vi "UHR-Fleezers Control (host) -Leonardo 04-2018 V4_fish.vi"(0 "Tab Green FB":T5(tab)=enum."Trap Control (RF)") -> ()   [LabVIEW 2014] (continued)
  n85 = xnode "Read/Write Control"("FPGA VI Reference In"=w153, "error in"=w173, "ai count"="AI Count (ticks)", "Interlace ON/OFF"=w139, "Number Interlace Cycles"=w138, "Set 1"=w19, "Set 2"=w18, "Set 3"=w17, "FB On/Off Set 1"=w260, "FB On/Off Set 2"=w259, "Interlace Off Parameters"=w137, "FB Setpoint Set 1"=w251, "FB Setpoint Set 2"=w250, "FB Gains"="PID gains", "FB output range"=cluster{"output high":i16, "output low":i16} {"output high"=3000, "output low"=0} ("FB output range 1"), "Cycles per step"=w236, "Scan BD"=w248, "Number of scans"=w232, "Scan steps"=w237, "Scan freq.  increment"=w238, "AO1 (Y)"=w220, "AO2 (X)"=w219, "Scan freq.  increment (MCL)"=w213, "Scan steps (MCL)"=w212, "Cycles per step (MCL)"=w211, "Number of scans (MCL)"=w210, "MCL count"=w136, "Cont. Scan (MCL)"=w209, "MCL Scan Axis"=w203, "1D or 2D Scan?"=w156, "N of AI1 Int Acq Sets"=w193, "BD 1 Delay (ticks)"="Freq switch delay", "Amp switch delay"="Amp switch delay", "Swap F1 and F2"="Swap F1 and F2", "APD Acq Rate Count"=w161, "APD to FIFO"=FALSE, "APD Gate Operating Mode"="APD Gate", "APD Gate ON Count"="APD Gate ON Count", "APD Gate OFF Count"="APD Gate OFF Count", "Invert APD Gate"="Invert APD Gate", "DIO count 1 (ticks)"="DIO count 1 (ticks)", "DIO count 2 (ticks)"="DIO count 2 (ticks)", "DIO count 3 (ticks)"="DIO count 3 (ticks)", "APD 1 AO scale factor"="APD 1 AO Mult.", "APD 2 AO scale factor"="APD 2 AO Mult.", "Diff FB Measurement?"=w24, "Dynamic Force FB (Ronen)"=w23, "Negate Diff?"=w22, "Next trap write delay (ticks)"="Next trap write delay (ticks)", "Phase offset method"="Phase offset method", "Phase Trap 1"="Phase increment trap 1", "RF phase reset before cycles"="RF phase reset before cycles", "Phase Trap 2"="Phase increment trap 2") -> ("FPGA VI Reference Out"=w131:T20, "error out"=w133:errorcluster)  [unwired: 1 in]
  n86 = local read "Green Laser ON/Interlacing"() -> (w134:bool)
  n87 = local read "Green laser mode"() -> (w135:enum32{"Laser ON", "Laser OFF", "Interlace"})
  n88 = local read "GI Frequency, OFF count"() -> (w127:u32)
  n89 = local read "GI Frequency, ON count"() -> (w126:u32)
  n90 = Multiply(x="Current When FB OFF (%)", y=655.35) -> (x*y=w117:dbl)
  n91 = local read "Green FB Count"() -> (w125:u32)
  n92 = Multiply(x="Green FB Setpoint (mV)", y=3.2767) -> (x*y=w114:dbl)
  n93 = To Unsigned Word Integer(number=w117) -> (unsigned 16bit integer=w115:u16)
  n94 = local read "Invert GI"() -> (w129:bool)
  n95 = To Word Integer(number=w114) -> (16bit integer=w112:i16)
  n96 = case shown="True" w134 {
    tunnel: w135 -> [_ w295]
    tunnel: [enum32{"Laser ON", "Laser OFF", "Interlace"}."Laser OFF" ("Green laser mode") w295] -> w128
    frame False {
    }
    frame True {
    }
  }
  n97 = local read "Trap Pos. AI1 X Pre-scale"() -> (w83:u16)
  n98 = local read "Trap Pos FB Monitor\nT1 or T2"() -> (w90:bool)
  n99 = local read "Trap Pos FB Int Count"() -> (w80:u16)
  n100 = local read "Trap Pos FB Negate Action"() -> (w89:bool)
  n101 = local read "Trap Pos. FB Offset Factor"() -> (w88:i64)
  n102 = local read "Trap Pos. FB Mult Factor"() -> (w87:i64)
  n103 = local read "Trap Pos. FB Gains"() -> (w85:T11)
  n104 = local read "Trap Pos. FB Range"() -> (w86:T12)
  n105 = xnode "Read/Write Control"("FPGA VI Reference In"=w131, "error in"=w133, "Green interlace ON count 2"=w126, "Green interlace OFF count 2"=w127, "Invert GI 2"=w129, "Operating Mode 2"=w128, "Green FB Gains"="Green FB Gains", "Green FB Setpoint"=w112, "Green FB On/Off"="Green FB On/Off", "Current Out"=w115, "Green int current ON count adj"="Green int current ON count adj", "Green FB Count"=w125, "Operating Mode"=w128, "Green interlace OFF count"=w127, "Green interlace ON count"=w126, "Invert GI"=w129, "Trap Pos FB Monitor T1 or T2"=w90, "Trap Pos FB Negate Action"=w89, "Trap Pos. FB Offset Factor"=w88, "Trap Pos. FB Mult Factor"=w87, "Trap pos. FB Range"=w86, "Trap Pos. FB Gains"=w85, "Force feedback"=FALSE, "AI1 X Scale"=w83, "Trap Pos to FIFO"=TRUE, "Trap Pos FB Int Count"=w80) -> ("FPGA VI Reference Out"=w130:T20, "error out"=w132:errorcluster)
  n106 = xnode "Invoke Method"("FPGA VI Reference In"=w130, "error in"=w132, "Requested Depth"="Trap AI FIFO Depth") -> ("FPGA VI Reference Out"=w93:T20, "error out"=w92:errorcluster)  [unwired: 1 out]
  n107 = xnode "Invoke Method"("FPGA VI Reference In"=w93, "error in"=w92, "Requested Depth"="Trap Position FIFO Depth") -> ("FPGA VI Reference Out"=w7:T20, "error out"=w5:errorcluster)  [unwired: 1 out]
  n108 = xnode "Invoke Method"("FPGA VI Reference In"=w7, "error in"=w5, "Requested Depth"="APD FIFO Depth (requires restart)") -> ("FPGA VI Reference Out"=w6:T20, "error out"=w4:errorcluster)  [unwired: 1 out]
  n109 = flat-sequence {
    tunnel: w154 -> [w300]
    tunnel: [w300] -> w153
    tunnel: [w296] -> w40
    tunnel: [w299] -> w152
    tunnel: [w298] -> w150
    tunnel: [w297] -> w151
    frame #0 {
      w297 = T16 {"Minimum"=60.0, "Maximum"=90.0, "Increment"=1.0} ("Min Max Inc")
      w298 = T16 {"Minimum"=0.0, "Maximum"=75.0, "Increment"=1.0} ("Data Entry Limits")
      w296 = T16 {"Minimum"=60.0, "Maximum"=90.0, "Increment"=1.0} ("Min Max Inc")
      w299 = T16 {"Minimum"=0.0, "Maximum"=75.0, "Increment"=1.0} ("Data Entry Limits")
      n110 = property on="BD 2 Frequency 1 (MHz)" class="DigNum (strict)"("Data Range"=w297) -> ()  [unwired: 2 in, 2 out]
      n111 = property on="BD 2 Frequency 3 (MHz)" class="DigNum (strict)"("Data Range"=w297) -> ()  [unwired: 2 in, 2 out]
      n112 = property on="BD 2 Frequency 2 (MHz)" class="DigNum (strict)"("Data Range"=w297) -> ()  [unwired: 2 in, 2 out]
      n113 = property on="BD 1 Frequency 1 (MHz)" class="DigNum (strict)"("Data Range"=w296) -> ()  [unwired: 2 in, 2 out]
      n114 = property on="BD 1 Frequency 2 (MHz)" class="DigNum (strict)"("Data Range"=w296) -> ()  [unwired: 2 in, 2 out]
      n115 = property on="BD 1 Frequency 3 (MHz)" class="DigNum (strict)"("Data Range"=w296) -> ()  [unwired: 2 in, 2 out]
      n116 = property on="BD 2 Amplitude 1 (%)" class="DigNum (strict)"("Data Range"=w298) -> ()  [unwired: 2 in, 2 out]
      n117 = property on="BD 2 Amplitude 2 (%)" class="DigNum (strict)"("Data Range"=w298) -> ()  [unwired: 2 in, 2 out]
      n118 = property on="BD 2 Amplitude 3 (%)" class="DigNum (strict)"("Data Range"=w298) -> ()  [unwired: 2 in, 2 out]
      n119 = property on="BD 1 Amplitude 3 (%)" class="DigNum (strict)"("Data Range"=w299) -> ()  [unwired: 2 in, 2 out]
      n120 = property on="BD 1 Amplitude 2 (%)" class="DigNum (strict)"("Data Range"=w299) -> ()  [unwired: 2 in, 2 out]
      n121 = property on="BD 1 Amplitude 1 (%)" class="DigNum (strict)"("Data Range"=w299) -> ()  [unwired: 2 in, 2 out]
      "X RF Frequency Limits (MHz)" <- w296
      "X RF Amplitude Limits (%)" <- w299
      "Y RF Amplitude Limits (%)" <- w298
      "Y RF Frequency Limits (MHz)" <- w297
    }
  }
  n122 = xnode "Invoke Method"("FPGA VI Reference In"=w6, "error in"=w4) -> ("FPGA VI Reference Out"=w60:T20, "error out"=w59:errorcluster)  [unwired: 1 in]
  n123 = flat-sequence "Initial FPGA Loop Relative Phase Adjustment" {
    tunnel: "Initial Phase Adjustment (APD 2 Gate)" -> [w302]
    tunnel: "Initial Phase Adjustment (GI) 2" -> [w303]
    tunnel: "Initial Phase Adj. (MCL)" -> [w304]
    tunnel: w59 -> [w305]
    tunnel: w60 -> [w306]
    tunnel: "Initial Phase Adjustment (GI)" -> [w307]
    tunnel: "Initial Phase Adjustment (AI1)" -> [w308]
    tunnel: [w308] -> w69
    tunnel: [w307] -> w68
    tunnel: [w306] -> w67
    tunnel: [w305] -> w66
    tunnel: [w304] -> w65
    tunnel: [w303] -> w64
    tunnel: [w302] -> w63
    tunnel: [w320] -> w179
    tunnel: [w314] -> w177
    tunnel: "Initial Phase Adjustment (APD Acq)" -> [w313]
    tunnel: "Initial Phase Adjustment (APD 1 Gate)" -> [w312]
    tunnel: "Initial Phase Adjustment (Green FB)" -> [w311]
    tunnel: w69 -> [w319]
    tunnel: w68 -> [w318]
    tunnel: w67 -> [w317]
    tunnel: w66 -> [w316]
    tunnel: w65 -> [w315]
    tunnel: w64 -> [w310]
    tunnel: w63 -> [w309]
    tunnel: w179 -> [w322]
    tunnel: [w323] -> w178
    tunnel: w177 -> [w323]
    tunnel: [w322] -> w176
    tunnel: w178 -> [w326]
    tunnel: w176 -> [w325]
    tunnel: [w328] -> w175
    tunnel: [w327] -> w174
    tunnel: [w330] -> w58
    tunnel: [w331] -> w61
    tunnel: w175 -> [w331]
    tunnel: w174 -> [w330]
    frame #0 {
      n124 = Wait (ms)(milliseconds to wait=u32 1000) -> ()  [unwired: 1 out]
    }
    frame #1 {
      n125 = xnode "Read/Write Control"("FPGA VI Reference In"=w317, "error in"=w316, "Phase count adjustment"=w319, "Phase count adjustment (GI)"=w318, "Phase count adjustment (MCL)"=w315, "Phase Count Adjustment (APD Acq)"=w313, "Phase count adjustment (APD 1 Gate)"=w312, "Phase count adjustment (APD 2 Gate)"=w309, "Phase count adjustment (Green FB)"=w311, "Phase count adjustment (GI) 2"=w310) -> ("FPGA VI Reference Out"=w314:T20, "error out"=w320:errorcluster)
    }
    frame #2 {
      n126 = Wait (ms)(milliseconds to wait=u32 1000) -> ()  [unwired: 1 out]
    }
    frame #3 {
      w324 = TRUE
      n127 = xnode "Read/Write Control"("FPGA VI Reference In"=w326, "error in"=w325, "+ phase"=w324, "+ phase (GI)"=w324, "+ phase (MCL)"=w324, "+ phase (APD Acq)"=w324, "+ phase (APD 1 Gate)"=w324, "+ phase (APD 2 Gate)"=w324, "+ phase (Green FB)"=w324, "+ phase (GI) 2"=w324) -> ("FPGA VI Reference Out"=w327:T20, "error out"=w328:errorcluster)
    }
    frame #4 {
      n128 = Wait (ms)(milliseconds to wait=u32 1000) -> ()  [unwired: 1 out]
    }
  }
  n129 = Unbundle By Name(w40) -> ("Minimum"=w39:dbl, "Maximum"=w38:dbl)
  n130 = local read "Phase adj. (Green FB)"() -> (w148:i16)
  n131 = local read "Phase adj. (GI) 2"() -> (w118:i16)
  n132 = local read "Phase adjust (MCL)"() -> (w204:i16)
  n133 = local read "Phase adj. (AI1)"() -> (w206:i16)
  n134 = local read "Phase adj. (GI)"() -> (w205:i16)
  n135 = Multiply(x=w39, y=w37) -> (x*y=w35:dbl)
  n136 = Multiply(x=w38, y=w37) -> (x*y=w36:dbl)
  n137 = Multiply(x=49152000.0, y=6.0) -> (x*y=w29:dbl)
  n138 = Scale By Power Of 2(n=w34, x=w35) -> (x*2^n=w31:dbl)
  n139 = Scale By Power Of 2(n=w34, x=w36) -> (x*2^n=w30:dbl)
  n140 = xnode "Read/Write Control"("FPGA VI Reference In"=w58, "error in"=w61, "Phase count adjustment"=w206, "Phase count adjustment (GI)"=w205, "Phase count adjustment (MCL)"=w204, "Phase Count Adjustment (APD Acq)"="Phase Adj. (APD Acq)", "Phase count adjustment (APD 1 Gate)"="Phase Adj. (APD 1 Gate)", "Phase count adjustment (APD 2 Gate)"="Phase Adj. (APD 2 Gate)", "Phase count adjustment (Green FB)"=w148, "Phase count adjustment (GI) 2"=w118) -> ("FPGA VI Reference Out"=w15:T20, "error out"=w14:errorcluster)
  n141 = Divide(x=w30, y=w29) -> (x/y=w27:dbl)
  n142 = Divide(x=w31, y=w29) -> (x/y=w28:dbl)
  n143 = To Unsigned Quad Integer(1:w28) -> (0:w26:u64)
  n144 = To Unsigned Quad Integer(1:w27) -> (0:w25:u64)
  n145 = xnode "Read/Write Control"("FPGA VI Reference In"=w15, "FB Min frequency"=w26, "FB Max Frequency"=w25) -> ()  [unwired: 1 in, 2 out]
  n146 = call "set RF board frequency - interlace.vi"("Board 2 Frequency Limits"=w151, "Board 1 Frequency Limits"=w40, "error in"=w14, "FPGA VI Reference In"=w15, "Board 2 Frequency 3 (MHz)"="BD 2 Frequency 3 (MHz)", "Board 1 Frequency 3 (MHz)"="BD 1 Frequency 3 (MHz)", "Board 2 Frequency 2 (MHz)"="BD 2 Frequency 2 (MHz)", "Board 2 Frequency 1 (MHz)"="BD 2 Frequency 1 (MHz)", "Board 1 Frequency 2 (MHz)"="BD 1 Frequency 2 (MHz)", "Board 1 Frequency 1  (MHz)"="BD 1 Frequency 1 (MHz)") -> ("error out"=w271:errorcluster, "FPGA VI Reference Out"=w272:T20)
  n147 = call "set RF board amplitude - interlace.vi"("Board 2 Amplitude Limits"=w150, "Board 1 Amplitude Limits"=w152, "error in"=w271, "FPGA VI Reference In"=w272, "Board 2 Amplitude 3 (%)"="BD 2 Amplitude 3 (%)", "Board 1 Amplitude 3 (%)"="BD 1 Amplitude 3 (%)", "Board 2 Amplitude 2 (%)"="BD 2 Amplitude 2 (%)", "Board 2 Amplitude 1 (%)"="BD 2 Amplitude 1 (%)", "Board 1 Amplitude 2 (%)"="BD 1 Amplitude 2 (%)", "Board 1 Amplitude 1 (%)"="BD 1 Amplitude 1 (%)") -> ("error out"=w56:errorcluster, "FPGA VI Reference Out"=w57:T20)
  n148 = flat-sequence {
    tunnel: w57 -> [w333]
    tunnel: w56 -> [w332]
    tunnel: [w333] -> w264
    tunnel: [w332] -> w263
    tunnel: [w341] -> w262
    tunnel: w264 -> [w341]
    tunnel: [w340] -> w261
    tunnel: w263 -> [w340]
    tunnel: w262 -> [w344]
    tunnel: w261 -> [w343]
    tunnel: [w344] -> w52
    tunnel: [w343] -> w51
    tunnel: [w350] -> w77
    tunnel: [w354] -> w62
    tunnel: w52 -> [w354]
    tunnel: w51 -> [w349]
    frame #0 {
      n149 = local read "Trap 1 (ON/OFF)"() -> (w334:bool)
      n150 = local write "Saving..."(FALSE ("Saving Data")) -> ()
      n151 = local write "Stop All"(FALSE ("Stop All")) -> ()
      n152 = local write "Index"(1.0 ("Index")) -> ()
      n153 = property on="Trap 1 ON" class="Bool (strict)"("Value"=w334) -> ()  [unwired: 2 in, 2 out]
      "Manipulating Trap" <- FALSE ("Manipulating Trap")
    }
    frame #1 {
      n154 = local read "Trap 2 (ON/OFF)"() -> (w339:bool)
      n155 = Wait (ms)(milliseconds to wait=u32 50) -> ()  [unwired: 1 out]
      n156 = property on="Trap 2 ON" class="Bool (strict)"("Val(Sgnl)"=w339) -> ()  [unwired: 2 in, 2 out]
    }
    frame #2 {
      n157 = local read "Scan Range (nm)"() -> (w345:dbl)
      n158 = call "Update messages.vi"("Message to add"="UHR-Fleezers ready.", "Old message string"="") -> ("New message string"=w348:string)
      n159 = local write "Messages"(w348) -> ()
      n160 = property on="Scan Range (nm)" class="DigNum (strict)"("Val(Sgnl)"=w345) -> ()  [unwired: 2 in, 2 out]
    }
    frame #3 {
      n161 = call "hamilton_controller.vi"("error in"=w349, "action"=T21."CONNECT") -> ("error out"=w351:errorcluster)  [unwired: 9 in]
      n162 = call "hamilton_controller.vi"("error in"=w351, "action"=T21."INITIALIZE VALVES") -> ("error out"=w350:errorcluster)  [unwired: 9 in]
    }
  }
  n163 = Subtract(x="BD 1 Frequency 1 (MHz)", y="BD 1 Frequency 2 (MHz)") -> (x-y=w192:dbl)
  n164 = Subtract(x="BD 2 Frequency 1 (MHz)", y="BD 2 Frequency 2 (MHz)") -> (x-y=w191:dbl)
  n165 = Square(x=w191) -> (x^2=w189:dbl)
  n166 = Square(x=w192) -> (x^2=w190:dbl)
  n167 = Add(x=w190, y=w189) -> (x+y=w188:dbl)
  n168 = Square Root(x=w188) -> (sqrt(x)=w187:dbl)
  n169 = local write "Trap Delta (MHz)"(w187) -> ()
  n170 = call "IMAQ Create"("Image Name"="APD 1 Image", "Image Type"=w99) -> ("New Image"=w98:T3)  [unwired: 3 in, 1 out]
  n171 = call "IMAQ Create"("Image Name"="APD 2 Image", "Image Type"=w99) -> ("New Image"=w97:T3)  [unwired: 3 in, 1 out]
  n172 = call "IMAQ Create"("Image Name"="Det. X Image", "Image Type"=w99) -> ("New Image"=w96:T3)  [unwired: 3 in, 1 out]
  n173 = call "IMAQ Create"("Image Name"="Det. Y Image", "Image Type"=w99) -> ("New Image"=w95:T3)  [unwired: 3 in, 1 out]
  n174 = Bundle("New Image"=w98, "New Image"=w97, "New Image"=w96, "New Image"=w95) -> (w94:T22)  [unwired: 1 in]
  n175 = Current VI's Path() -> (path=w41:path)
  n176 = Concatenate Strings("N.D.", "\r\n") -> (w45:string)
  n177 = Strip Path(path=w41) -> (stripped path=w42:path)  [unwired: 1 out]
  n178 = Initialize Array(w45, 4, 3) -> (w48:string[][])
  n179 = Build Path(base path=w42, name or relative path="Locations.txt") -> (appended path=→"Location path":path)
  n180 = local write "Location Matrix"(w48) -> ()
  n181 = while {
    stop <- w355 stop-if-true
    n182 = event shown="[0] Timeout" {
      selector: _ -> [_ _ _ _ _ _ _ _ _]
      dyn-events: _ -> [_ _ _ _ _ _ _ _ _]
      timeout: 10 -> [_ _ _ _ _ _ _ _ _]
      tunnel: [FALSE _ _ _ _ _ _ _ TRUE] -> w355
      event Timeout {
        # "Change the trajectory mode to Jog"
        # "Query and display stage positions"
        # "Setting ESP300 left and right limits for Z-axis, input in mm"
        # "Display Selected Location"
        n183 = event-data() -> ()  [unwired: 1 in, 2 out]
        n184 = local read "Capture Locations"() -> (w380:i32)
        n185 = local read "Location Matrix"() -> (w381:string[][])
        n186 = Concatenate Strings("1TP;\n2TP;\n3TP;\n1MD?;\n2MD?;\n3MD?" ("Substring"), "\r") -> (w364:string)
        n187 = local read "ESP Port"() -> (w367:refnum<visa-resource-name>)
        n188 = Index Array(array=w381, index (row)=w380) -> (element=w379:string[])  [unwired: 1 in]
        n189 = local read "ESP Port"() -> (w376:refnum<visa-resource-name>)
        n190 = VISA Write(VISA resource name=w367, write buffer=w364, error in (no error)="error in") -> (VISA resource name out=w365:refnum<visa-resource-name>, error out=w363:errorcluster)  [unwired: 1 out]
        n191 = Concatenate Strings("3SL" ("Substring"), "ESP ZL-Limit", ";3SR", "ESP ZR-Limit", "\r") -> (w375:string)
        n192 = Array To Cluster(array=w379) -> (cluster=w378:T23)
        n193 = case shown="True" TRUE ("Case Constant\n(See Context Help)") {
          tunnel: w365 -> [_ w419]
          tunnel: w363 -> [w400 w418]
          tunnel: [w400 w402] -> w369
          frame False {
          }
          frame True {
            w412 = u16 10 items=["1.0"=10, "1.5"=15, "2.0"=20] ("Serial Settings:Stop Bits")
            w413 = u16 0 items=["None", "Odd", "Even", "Mark", "Space"] ("Serial Settings:Parity")
            n194 = property class="Instr"(reference=w419, error in=w418, "Baud"=u32 921600 ("Serial Settings:Baud Rate"), "Data Bits"=u16 8 ("Serial Settings:Data Bits"), "Parity"=w413, "Stop Bits"=w412) -> (reference out=w417:refnum<visa-resource-name>, error out=w416:errorcluster, "Bytes at Port"=w401:u32)
            n195 = Wait (ms)(milliseconds to wait=u32 10) -> ()  [unwired: 1 out]
            n196 = VISA Read(VISA resource name=w417, byte count=w401, error in (no error)=w416) -> (VISA resource name out=w425:refnum<visa-resource-name>, read buffer=→"X Pos":string, error out=w426:errorcluster)  [unwired: 1 out]
            n197 = VISA Read(VISA resource name=w425, byte count=w401, error in (no error)=w426) -> (VISA resource name out=w423:refnum<visa-resource-name>, read buffer=→"Y Pos":string, error out=w424:errorcluster)  [unwired: 1 out]
            n198 = VISA Read(VISA resource name=w423, byte count=w401, error in (no error)=w424) -> (VISA resource name out=w411:refnum<visa-resource-name>, read buffer=→"Z Pos Pos":string, error out=w410:errorcluster)  [unwired: 1 out]
            n199 = VISA Read(VISA resource name=w411, byte count=w401, error in (no error)=w410) -> (VISA resource name out=w407:refnum<visa-resource-name>, read buffer=→"X Motion":string, error out=w408:errorcluster)  [unwired: 1 out]
            n200 = VISA Read(VISA resource name=w407, byte count=w401, error in (no error)=w408) -> (VISA resource name out=w406:refnum<visa-resource-name>, read buffer=→"Y Motion":string, error out=w404:errorcluster)  [unwired: 1 out]
            n201 = VISA Read(VISA resource name=w406, byte count=w401, error in (no error)=w404) -> (read buffer=→"Z motion":string, error out=w402:errorcluster)  [unwired: 2 out]
          }
        }
        "error out" <- w369
        n202 = VISA Write(VISA resource name=w376, write buffer=w375) -> ()  [unwired: 1 in, 3 out]
        n203 = local write item#483(w378) -> ()
        n204 = disable-structure shown="Disabled" {
          frame Disabled {
            # "Change Low Jog Velocity"
            # "Change High Jog Velocity"
            n205 = Concatenate Strings("1JH" ("Substring"), "Axis 1", "2JH" ("Substring"), "Axis 2", "3JH" ("Substring"), "Axis 3", "\r") -> (w399:string)
            n206 = local read "ESP Port"() -> (w398:refnum<visa-resource-name>)
            n207 = VISA Write(VISA resource name=w398, write buffer=w399) -> ()  [unwired: 1 in, 3 out]
            n208 = Concatenate Strings("1JW" ("Substring"), "Axis 1", "2JW" ("Substring"), "Axis 2", "3JW" ("Substring"), "Axis 3", "\r") -> (w390:string)
            n209 = local read "ESP Port"() -> (w389:refnum<visa-resource-name>)
            n210 = VISA Write(VISA resource name=w389, write buffer=w390) -> ()  [unwired: 1 in, 3 out]
          }
          frame Enabled {
          }
        }
        n211 = local read "ESP Port"() -> (w357:refnum<visa-resource-name>)
        n212 = Concatenate Strings("1TJ3;\n2TJ3;\n3TJ3" ("Substring"), "\r") -> (w358:string)
        n213 = VISA Write(VISA resource name=w357, write buffer=w358) -> ()  [unwired: 1 in, 3 out]
      }
      event "Goto Top (F6)": Value Change {
        n214 = event-data() -> ()  [unwired: 1 in, 5 out]
        n215 = stacked-sequence {
          frame #0 {
            # "stop motions of all axes before going to avoid reversing of direction"
            n216 = local read "ESP Port"() -> (w431:refnum<visa-resource-name>)
            n217 = Concatenate Strings("ST" ("Substring"), "\r") -> (w428:string)
            n218 = VISA Write(VISA resource name=w431, write buffer=w428) -> ()  [unwired: 1 in, 3 out]
          }
          frame #1 {
            n219 = Wait (ms)(milliseconds to wait=u32 50) -> ()  [unwired: 1 out]
          }
          frame #2 {
            # "Change the trajectory mode to Trapezoidal"
            n220 = local read "ESP Port"() -> (w436:refnum<visa-resource-name>)
            n221 = Concatenate Strings("1TJ1;\n2TJ1;\n3TJ1" ("Substring"), "\r") -> (w433:string)
            n222 = VISA Write(VISA resource name=w436, write buffer=w433) -> ()  [unwired: 1 in, 3 out]
          }
          frame #3 {
            # "Go to Top Dispensor"
            n223 = local read "Location Matrix"() -> (w448:string[][])
            n224 = Index Array(array=w448, index (row)=0) -> (element=w444:string[])  [unwired: 1 in]
            n225 = Decimate 1D Array(w444) -> (w442:string[], w440:string[], w438:string[])
            n226 = local read "ESP Port"() -> (w445:refnum<visa-resource-name>)
            n227 = Concatenate Strings("1PA" ("Substring"), w442, "2PA" ("Substring"), w440, "3PA" ("Substring"), w438, "\r") -> (w446:string)
            n228 = VISA Write(VISA resource name=w445, write buffer=w446) -> ()  [unwired: 1 in, 3 out]
          }
          frame #4 {
            n229 = Wait (ms)(milliseconds to wait=u32 100) -> ()  [unwired: 1 out]
          }
          frame #5 {
            # "Change the trajectory mode to Jog"
            n230 = local read "ESP Port"() -> (w453:refnum<visa-resource-name>)
            n231 = Concatenate Strings("1TJ3;\n2TJ3;\n3TJ3" ("Substring"), "\r") -> (w450:string)
            n232 = VISA Write(VISA resource name=w453, write buffer=w450) -> ()  [unwired: 1 in, 3 out]
          }
        }
      }
      event "Goto Exp (F8)": Value Change {
        n233 = event-data() -> ()  [unwired: 1 in, 5 out]
        n234 = stacked-sequence {
          frame #0 {
            # "stop motions of all axes before going to avoid reversing of direction"
            n235 = local read "ESP Port"() -> (w457:refnum<visa-resource-name>)
            n236 = Concatenate Strings("ST" ("Substring"), "\r") -> (w454:string)
            n237 = VISA Write(VISA resource name=w457, write buffer=w454) -> ()  [unwired: 1 in, 3 out]
          }
          frame #1 {
            n238 = Wait (ms)(milliseconds to wait=u32 50) -> ()  [unwired: 1 out]
          }
          frame #2 {
            # "Change the trajectory mode to Trapezoidal"
            n239 = local read "ESP Port"() -> (w462:refnum<visa-resource-name>)
            n240 = Concatenate Strings("1TJ1;\n2TJ1;\n3TJ1" ("Substring"), "\r") -> (w459:string)
            n241 = VISA Write(VISA resource name=w462, write buffer=w459) -> ()  [unwired: 1 in, 3 out]
          }
          frame #3 {
            # "Go to Experimental"
            n242 = local read "Location Matrix"() -> (w474:string[][])
            n243 = Index Array(array=w474, index (row)=2) -> (element=w470:string[])  [unwired: 1 in]
            n244 = Decimate 1D Array(w470) -> (w468:string[], w466:string[], w464:string[])
            n245 = Concatenate Strings("1PA" ("Substring"), w468, "2PA" ("Substring"), w466, "3PA" ("Substring"), w464, "\r") -> (w472:string)
            n246 = local read "ESP Port"() -> (w471:refnum<visa-resource-name>)
            n247 = VISA Write(VISA resource name=w471, write buffer=w472) -> ()  [unwired: 1 in, 3 out]
          }
          frame #4 {
            n248 = Wait (ms)(milliseconds to wait=u32 200) -> ()  [unwired: 1 out]
          }
          frame #5 {
            # "Change the trajectory mode to Jog"
            n249 = local read "ESP Port"() -> (w476:refnum<visa-resource-name>)
            n250 = Concatenate Strings("1TJ3;\n2TJ3;\n3TJ3" ("Substring"), "\r") -> (w479:string)
            n251 = VISA Write(VISA resource name=w476, write buffer=w479) -> ()  [unwired: 1 in, 3 out]
          }
        }
      }
      event "Goto Bottom (F7)": Value Change {
        n252 = event-data() -> ()  [unwired: 1 in, 5 out]
        n253 = stacked-sequence {
          frame #0 {
            # "stop motions of all axes before going to avoid reversing of direction"
            n254 = local read "ESP Port"() -> (w483:refnum<visa-resource-name>)
            n255 = Concatenate Strings("ST" ("Substring"), "\r") -> (w480:string)
            n256 = VISA Write(VISA resource name=w483, write buffer=w480) -> ()  [unwired: 1 in, 3 out]
          }
          frame #1 {
            n257 = Wait (ms)(milliseconds to wait=u32 50) -> ()  [unwired: 1 out]
          }
          frame #2 {
            # "Change the trajectory mode to Trapezoidal"
            n258 = local read "ESP Port"() -> (w488:refnum<visa-resource-name>)
            n259 = Concatenate Strings("1TJ1;\n2TJ1;\n3TJ1" ("Substring"), "\r") -> (w485:string)
            n260 = VISA Write(VISA resource name=w488, write buffer=w485) -> ()  [unwired: 1 in, 3 out]
          }
          frame #3 {
            # "Go to Bottom Dispensor"
            n261 = local read "Location Matrix"() -> (w500:string[][])
            n262 = Index Array(array=w500, index (row)=1) -> (element=w496:string[])  [unwired: 1 in]
            n263 = Decimate 1D Array(w496) -> (w494:string[], w492:string[], w490:string[])
            n264 = Concatenate Strings("1PA" ("Substring"), w494, "2PA" ("Substring"), w492, "3PA" ("Substring"), w490, "\r") -> (w498:string)
            n265 = local read "ESP Port"() -> (w497:refnum<visa-resource-name>)
            n266 = VISA Write(VISA resource name=w497, write buffer=w498) -> ()  [unwired: 1 in, 3 out]
          }
          frame #4 {
            n267 = Wait (ms)(milliseconds to wait=u32 200) -> ()  [unwired: 1 out]
          }
          frame #5 {
            # "Change the trajectory mode to Jog"
            n268 = local read "ESP Port"() -> (w502:refnum<visa-resource-name>)
            n269 = Concatenate Strings("1TJ3;\n2TJ3;\n3TJ3" ("Substring"), "\r") -> (w505:string)
            n270 = VISA Write(VISA resource name=w502, write buffer=w505) -> ()  [unwired: 1 in, 3 out]
          }
        }
      }
      event "Capture": Value Change {
        n271 = event-data() -> ()  [unwired: 1 in, 5 out]
        n272 = local read "Capture Locations"() -> (w506:i32)
        n273 = local read "Z Pos Pos"() -> (w507:string)
        n274 = local read "X Pos"() -> (w509:string)
        n275 = local read "Y Pos"() -> (w508:string)
        n276 = case shown="1" w506 {
          selector: w506 -> [w513 w520 w527 w534]
          tunnel: w509 -> [w516 w523 w530 w537]
          tunnel: w508 -> [w515 w522 w529 w536]
          tunnel: w507 -> [w514 w521 w528 w535]
          frame 0, Default {
            # "Capture Top Dispensor Location"
            n277 = local read "Location Matrix"() -> (w512:string[][])
            n278 = Build Array(w516, w515, w514) -> (w511:string[])
            n279 = Replace Array Subset(array=w512, new element=w511, index (row)=w513) -> (w510:string[][])  [unwired: 1 in]
            n280 = local write "Location Matrix"(w510) -> ()
          }
          frame 1 {
            # "Capture Bottom Dispensor Location"
            n281 = local read "Location Matrix"() -> (w519:string[][])
            n282 = Build Array(w523, w522, w521) -> (w518:string[])
            n283 = Replace Array Subset(array=w519, new element=w518, index (row)=w520) -> (w517:string[][])  [unwired: 1 in]
            n284 = local write "Location Matrix"(w517) -> ()
          }
          frame 2 {
            # "Capture Experimental Region Location"
            n285 = local read "Location Matrix"() -> (w526:string[][])
            n286 = Build Array(w530, w529, w528) -> (w525:string[])
            n287 = Replace Array Subset(array=w526, new element=w525, index (row)=w527) -> (w524:string[][])  [unwired: 1 in]
            n288 = local write "Location Matrix"(w524) -> ()
          }
          frame 3 {
            # "Capture Other Location"
            n289 = local read "Location Matrix"() -> (w533:string[][])
            n290 = Build Array(w537, w536, w535) -> (w532:string[])
            n291 = Replace Array Subset(array=w533, new element=w532, index (row)=w534) -> (w531:string[][])  [unwired: 1 in]
            n292 = local write "Location Matrix"(w531) -> ()
          }
        }
      }
      event "Save": Value Change {
        # "reshape Location Matrix to 1-D array to write"
        n293 = event-data() -> ()  [unwired: 1 in, 5 out]
        n294 = local read "Location Matrix"() -> (w541:string[][])
        n295 = local read "Location path"() -> (w538:path)
        n296 = Reshape Array(w541, 12) -> (w539:string[])
        n297 = Write to Text File(file (use dialog)=w538, text=w539) -> ()  [unwired: 2 in, 3 out]
      }
      event "VISA Clear": Value Change {
        n298 = event-data() -> ()  [unwired: 1 in, 5 out]
        n299 = local read "ESP Port"() -> (w542:refnum<visa-resource-name>)
        n300 = VISA Clear(VISA resource name=w542) -> ()  [unwired: 1 in, 2 out]
      }
      event "Activate Joystick": Value Change {
        # "Change the trajectory mode to Jog"
        n301 = event-data() -> ()  [unwired: 1 in, 5 out]
        n302 = disable-structure shown="Disabled" {
          frame Disabled {
            n303 = case shown="True" "Activate Joystick" {
              frame False {
              }
              frame True {
                # "Change the trajectory mode to Jog"
                n304 = local read "ESP Port"() -> (w551:refnum<visa-resource-name>)
                n305 = Concatenate Strings("1TJ3;\n2TJ3;\n3TJ3" ("Substring"), "\r") -> (w548:string)
                n306 = VISA Write(VISA resource name=w551, write buffer=w548) -> ()  [unwired: 1 in, 3 out]
              }
            }
          }
          frame Enabled {
          }
        }
        n307 = local read "ESP Port"() -> (w543:refnum<visa-resource-name>)
        n308 = Concatenate Strings("1TJ3;\n2TJ3;\n3TJ3" ("Substring"), "\r") -> (w546:string)
        n309 = VISA Write(VISA resource name=w543, write buffer=w546) -> ()  [unwired: 1 in, 3 out]
      }
      event "Stop All": Mouse Down {
        n310 = event-data() -> ()  [unwired: 1 in, 5 out]
      }
    }
  }
  n311 = disable-structure shown="Disabled" {
    disable-tunnel: w62 -> [w581 _]
    frame Disabled {
      w576 = T17 0 items=["Grayscale (U8)", "Grayscale (I16)", "Grayscale (SGL)", "Complex (CSG)", "RGB (U32)", "HSL (U32)", "RGB (U64)", "Grayscale (U16)"] ("Image Type")
      n312 = call <vilib>:"IMAQ Init.vi"("Interface Name"="img0") -> ("error out"=w578:errorcluster, "IMAQ Session Out"=w580:refnum<k11>)  [unwired: 9 in]
      n313 = call <vilib>:"IMAQ Grab Setup.vi"("error in (no error)"=w578, "IMAQ Session In"=w580) -> ("error out"=w574:errorcluster, "IMAQ Session Out"=w575:refnum<k11>)  [unwired: 8 in]
      n314 = call "IMAQ Create"("Image Name"="untitled", "Image Type"=w576) -> ("New Image"=w573:T3)  [unwired: 3 in, 1 out]
      n315 = call <vilib>:"Application Directory.vi"() -> ("Application Directory"=w560:path)
      n316 = Build Path(base path=w560, name or relative path="_trap_screen_positions") -> (appended path=w568:path)
      n317 = Open/Create/Replace File(file path (use dialog)=w568, operation (0:open)=T24."open or create", access (0:read/write)=enum16{"read/write", "read-only", "write-only"}."read/write") -> (refnum out=w570:refnum<file>)  [unwired: 3 in, 2 out]
      n318 = local read "Trap Sets"() -> (w562:u32)
      n319 = for "Load trap positions on video screen from file." {
        N: w562 -> [_]
        tunnel: [w588] -> w563
        tunnel: w570 -> [w587]
        tunnel: [w584] -> w559 mode=indexing
        w586 = 4
        n320 = for {
          N: w586 -> [_]
          tunnel: [w592] -> w588
          tunnel: w587 -> [w591]
          tunnel: w586 -> [w590]
          tunnel: [w589] -> w585 mode=indexing
          n321 = Read from Binary File(5:w590, 11:w591) -> (2:w589:i32, 3:w592:refnum<file>)  [unwired: 4 in, 2 out]
        }
        n322 = Array To Cluster(array=w585) -> (cluster=w584:T28)
      }
      n323 = node-c288() -> (w583:T25)  [unwired: 4 in]
      n324 = timed-loop "acquire video and stage position" {
        timing: w583 -> [_]
        timing-out: [_] -> w582
        tunnel: w575 -> [w611]
        tunnel: w574 -> [w610]
        tunnel: w573 -> [w609]
        tunnel: [w608] -> w555
        tunnel: [w605] -> w556
        tunnel: [w606] -> w554
        tunnel: w581 -> [_]
        shift-right: [w602] -> w572
        shift-left: w559 -> [w603]
        tunnel: w562 -> [w600]
        stop <- w607 stop-if-true
        n325 = node-c288() -> ()  [unwired: 1 in, 1 out]
        n326 = event shown="[1] \"Stop All\": Value Change" {
          selector: _ -> [_ _ _ _]
          dyn-events: _ -> [_ _ _ _]
          timeout: 10 -> [_ _ _ _]
          tunnel: w611 -> [w622 w637 w646 w665]
          tunnel: w610 -> [w621 w639 w644 w667]
          tunnel: w609 -> [w620 w638 w645 w666]
          tunnel: [w619 w637 w646 w665] -> w608
          tunnel: [w612 w641 FALSE FALSE] -> w607
          tunnel: [w616 w639 w644 w667] -> w606
          tunnel: [w615 w638 w645 w666] -> w605
          tunnel: "radius" -> [_ _ w651 _]
          tunnel: w603 -> [w613 w640 w649 _]
          tunnel: [w613 w640 w650 cluster{i32, i32, i32, i32}[] []] -> w602
          tunnel: w600 -> [_ _ w642 _]
          event Timeout {
            n327 = event-data() -> ()  [unwired: 1 in, 2 out]
            n328 = call <vilib>:"IMAQ Grab Acquire.vi"("error in (no error)"=w621, "Image In"=w620, "IMAQ Session In"=w622) -> ("error out"=w617:errorcluster, "Image Out"=w618:T3, "IMAQ Session Out"=w619:refnum<k11>)  [unwired: 5 in, 1 out]
            n329 = case shown="True" "trap\nmarkers?" {
              tunnel: w613 -> [_ w630]
              tunnel: w618 -> [w624 w629]
              tunnel: w617 -> [w623 w628]
              tunnel: [w623 w627] -> w616
              tunnel: [w624 w625] -> w615
              frame False {
              }
              frame True {
                n330 = for {
                  tunnel: w630 -> [w636] mode=indexing
                  shift-right: [w634] -> w625
                  shift-left: w629 -> [w635]
                  tunnel: w628 -> [w633]
                  tunnel: [w632] -> w627
                  tunnel: u32 16711680 ("Color") -> [w631]
                  n331 = call "IMAQ Overlay Oval"("Color"=w631, "error in (no error)"=w633, "Bounding Rectangle"=w636, "Image"=w635) -> ("error out"=w632:errorcluster, "Image Out"=w634:T3)  [unwired: 6 in]
                }
              }
            }
            "Primary Video Display" <- w615
            n332 = Unbundle By Name(w617) -> ("status"=w612:bool)
          }
          event "Stop All": Value Change {
            n333 = event-data() -> ()  [unwired: 1 in, 5 out]
            n334 = local read "Stop All"() -> (w641:bool)
          }
          event "Primary Video Display": Mouse Down {
            n335 = event-data() -> ()  [unwired: 1 in, 7 out]
            n336 = Array Size(array=w649) -> (size(s)=w648:i32)
            n337 = Less?(x=w648, y=w642) -> (x < y?=w647:bool)
            n338 = case shown="True" w647 {
              tunnel: w651 -> [_ w661]
              tunnel: w649 -> [w652 w655]
              tunnel: [w652 w654] -> w650
              frame False {
              }
              frame True {
                n339 = property on="Primary Video Display"() -> ("Last Mouse Position"=w653)  [unwired: 2 in, 2 out]
                n340 = Unbundle By Name(w653) -> ("X"=w663, "Y"=w662)
                n341 = Add(x=w662, y=w661) -> (x+y=w659:i32)
                n342 = Subtract(x=w662, y=w661) -> (x-y=w657:i32)
                n343 = Add(x=w663, y=w661) -> (x+y=w658:i32)
                n344 = Subtract(x=w663, y=w661) -> (x-y=w660:i32)
                n345 = Bundle(w660, w659, w658, w657) -> (w656:cluster{i32, i32, i32, i32})  [unwired: 1 in]
                n346 = Build Array (concatenate)(w655, w656) -> (w654:T29)
              }
            }
          }
          event "clear markers": Value Change {
            n347 = event-data() -> ()  [unwired: 1 in, 5 out]
          }
        }
        n348 = node-c288() -> ()  [unwired: 1 in, 1 out]
      }
      n349 = node-c288(w582) -> ()  [unwired: 1 out]
      n350 = Set File Position(offset (in bytes) (0)=i64 0, refnum=w563, from (0:start)=enum16{"start", "end", "current"}."start") -> (refnum out=w564:refnum<file>)  [unwired: 1 in, 1 out]
      n351 = for "Write trap positions to file so they can be remembered\nwhen program is removed from memory" {
        tunnel: w572 -> [w596] mode=indexing
        tunnel: [w594] -> w571
        tunnel: w564 -> [w593]
        n352 = Cluster To Array(cluster=w596) -> (array=w595:i32[])
        n353 = for {
          tunnel: w595 -> [w599] mode=indexing
          tunnel: [w598] -> w594
          tunnel: w593 -> [w597]
          n354 = Write to Binary File(file (use dialog)=w597, data=w599) -> (refnum out=w598:refnum<file>)  [unwired: 4 in, 2 out]
        }
      }
      n355 = Close File(refnum=w571) -> ()  [unwired: 1 in, 2 out]
      n356 = call "IMAQ Dispose"("Image"=w556, "error in (no error)"=w554) -> ("error out"=w553:errorcluster)  [unwired: 4 in]
      n357 = call <vilib>:"IMAQ Stop.vi"("error in (no error)"=w553, "IMAQ Session In"=w555) -> ("error out"=w557:errorcluster, "IMAQ Session Out"=w558:refnum<k11>)  [unwired: 8 in]
      n358 = call <vilib>:"IMAQ Close.vi"("error in (no error)"=w557, "IMAQ Session In"=w558) -> ()  [unwired: 9 in, 1 out]
    }
    frame Enabled {
    }
  }
  n359 = disable-structure shown="Enabled" {
    disable-tunnel: [w674 _] -> w72
    disable-tunnel: w62 -> [w673 _]
    frame Enabled {
      n360 = node-c288() -> (w676:T25)  [unwired: 4 out]
      n361 = timed-loop "Rough control of MCL mirror stage (debugging)" {
        tunnel: w673 -> [w679]
        tunnel: [w678] -> w674
        timing: w676 -> [_]
        timing-out: [_] -> w675
        stop <- w678 stop-if-true
        n362 = node-c288() -> ()  [unwired: 2 out]
        n363 = case shown="1" "MCL Mode" {
          tunnel: w679 -> [_ w682 w729]
          frame 0, Default {
            # "manual positioning"
          }
          frame 1 {
            # "sinusoidal wave"
            n364 = node-c288() -> (w684:T25)  [unwired: 4 out]
            n365 = timed-loop "Oscillate MCL mirror" {
              timing: w684 -> [_]
              timing-out: [_] -> w683
              tunnel: w682 -> [w723]
              i -> [w722]
              stop <- w685 stop-if-true
              n366 = node-c288() -> (w721:i64)  [unwired: 1 out]
              n367 = Multiply(x="AO1", y=32767.0) -> (x*y=w717:dbl)
              n368 = Multiply(x="AO2", y=32767.0) -> (x*y=w712:dbl)
              n369 = Divide(x=w717, y=10.0) -> (x/y=w718:dbl)
              n370 = Divide(x=w712, y=10.0) -> (x/y=w713:dbl)
              n371 = To Word Integer(number=w718) -> (16bit integer=w710:i16)
              n372 = To Word Integer(number=w713) -> (16bit integer=w709:i16)
              n373 = Divide(x=w721, y=i64 1000) -> (x/y=w692:dbl)
              n374 = Multiply(x=w692, y=w722) -> (x*y=w703:dbl)
              n375 = Multiply(x="Osc. freq. (Hz) 2", y=6.283185307179586) -> (x*y=w704:dbl)
              n376 = Multiply(x=w704, y=w703) -> (x*y=w702:dbl)
              n377 = Sine(x=w702) -> (sin(x)=w701:dbl)
              n378 = Multiply(x=w701, y="Osc. amp. (V)") -> (x*y=w699:dbl)
              n379 = Add(x=w699, y="Osc. center (V)") -> (x+y=w697:dbl)
              n380 = Divide(x=w697, y=10.0) -> (x/y=w695:dbl)
              n381 = Multiply(x=w695, y=32767.0) -> (x*y=w690:dbl)
              n382 = Select(t=w690, s="Scan axis", f=w710) -> (s? t:f=w708:dbl)
              n383 = Select(t=w709, s="Scan axis", f=w690) -> (s? t:f=w707:dbl)
              n384 = local read "MCL Mode"() -> (w689:u16)
              n385 = Not Equal?(x=w689, y=u16 1) -> (x != y?=w686:bool)
              n386 = local read "Stop All"() -> (w687:bool)
              n387 = xnode "Read/Write Control"("FPGA VI Reference In"=w723, "AO1 (Y)"=w708, "AO2 (X)"=w707) -> ()  [unwired: 1 in, 2 out]
              n388 = Compound Arithmetic op=OR(w687, w686) -> (w685:bool)
              n389 = node-c288() -> ()  [unwired: 2 out]
            }
            n390 = node-c288(w683) -> ()  [unwired: 1 out]
          }
          frame 2 {
            # "linear scan"
            n391 = case shown="True" "Start Scan" {
              tunnel: w729 -> [_ w741]
              frame False {
              }
              frame True {
                n392 = Subtract(x="End (V)", y="Begin (V)") -> (x-y=w737:dbl)
                n393 = Decrement(x="N Points") -> (x-1=w736:dbl)
                n394 = Divide(x=w737, y=w736) -> (x/y=w734:dbl)
                n395 = for {
                  N: "N Points" -> [_]
                  tunnel: "Begin (V)" -> [w754]
                  tunnel: w741 -> [w746]
                  tunnel: [w745] -> w740 mode=indexing
                  tunnel: w734 -> [w744]
                  tunnel: [w742] -> w733 mode=indexing
                  i -> [w753]
                  n396 = Multiply(x=w744, y=w753) -> (x*y=w752:dbl)
                  n397 = Add(x=w754, y=w752) -> (x+y=w749:dbl)
                  n398 = local read "Scan axis"() -> (w743:bool)
                  n399 = local read "AO1"() -> (w751:dbl)
                  n400 = local read "AO2"() -> (w750:dbl)
                  n401 = Select(t=w749, s=w743, f=w751) -> (s? t:f=w748:dbl)
                  n402 = Select(t=w750, s=w743, f=w749) -> (s? t:f=w747:dbl)
                  n403 = flat-sequence {
                    tunnel: w748 -> [w758]
                    tunnel: w747 -> [w757]
                    tunnel: w746 -> [w755]
                    tunnel: [w768] -> w745
                    tunnel: [w767] -> w742
                    frame #0 {
                      w761 = 10.0 ("y")
                      w756 = 32767.0 ("y")
                      n404 = Multiply(x=w758, y=w756) -> (x*y=w764:dbl)
                      n405 = Multiply(x=w757, y=w756) -> (x*y=w762:dbl)
                      n406 = Divide(x=w764, y=w761) -> (x/y=w765:dbl)
                      n407 = Divide(x=w762, y=w761) -> (x/y=w763:dbl)
                      n408 = To Word Integer(number=w765) -> (16bit integer=w759:i16)
                      n409 = To Word Integer(number=w763) -> (16bit integer=w760:i16)
                      n410 = xnode "Read/Write Control"("FPGA VI Reference In"=w755, "AO1 (Y)"=w759, "AO2 (X)"=w760) -> ()  [unwired: 1 in, 2 out]
                    }
                    frame #1 {
                      n411 = Wait (ms)(milliseconds to wait="DAQ Delay (ms)") -> ()  [unwired: 1 out]
                    }
                    frame #2 {
                      n412 = local read "Slow mean"() -> (w768:dbl)
                      n413 = local read "Sigma"() -> (w767:dbl)
                    }
                  }
                }
                n414 = Bundle("Begin (V)"="Begin (V)", w734, w740) -> (→"MCL Scan":cluster{"Begin (V)":dbl, dbl, dbl[]})  [unwired: 1 out]
                n415 = Bundle("Begin (V)"="Begin (V)", w734, w733) -> (→"MCL Scan 2":cluster{"Begin (V)":dbl, dbl, dbl[]})  [unwired: 1 out]
              }
            }
          }
        }
        n416 = local read "Stop All"() -> (w678:bool)
        n417 = node-c288() -> ()  [unwired: 2 out]
      }
      n418 = node-c288(w675) -> ()  [unwired: 1 out]
    }
    frame Disabled {
    }
  }
  n419 = node-c288(2 ("Processor")) -> (w55:T25)  [unwired: 3 in]
  n420 = timed-loop "Control parameters (event loop)" {
    tunnel: w62 -> [w774]
    shift-right: [w773] -> _
    shift-left: errorcluster {"status"=FALSE, "code"=0, "source"=""} ("error out") -> [w772]
    tunnel: [w771] -> w74
    timing: w55 -> [_]
    timing-out: [_] -> w54
    stop <- w771 stop-if-true
    n421 = node-c288() -> ()  [unwired: 1 in, 1 out]
    n422 = event shown="[54] \"Simulate stepping\": Value Change" {
      selector: _ -> [_ _ _ _ _ _ _ _ _ _ _ _ _ _ _ _ _ _ _ _ _ _ _ _ _ _ _ _ _ _ _ _ _ _ _ _ _ _ _ _ _ _ _ _ _ _ _ _ _ _ _ _ _ _ _ _ _ _ _ _ _ _]
      dyn-events: _ -> [_ _ _ _ _ _ _ _ _ _ _ _ _ _ _ _ _ _ _ _ _ _ _ _ _ _ _ _ _ _ _ _ _ _ _ _ _ _ _ _ _ _ _ _ _ _ _ _ _ _ _ _ _ _ _ _ _ _ _ _ _ _]
      timeout: _ -> [_ _ _ _ _ _ _ _ _ _ _ _ _ _ _ _ _ _ _ _ _ _ _ _ _ _ _ _ _ _ _ _ _ _ _ _ _ _ _ _ _ _ _ _ _ _ _ _ _ _ _ _ _ _ _ _ _ _ _ _ _ _]
      tunnel: w774 -> [w815 _ _ _ w852 _ w870 w876 _ _ _ _ w953 _ _ w997 w1003 w1007 w1012 w1048 w1066 w1073 w1091 w1102 w1113 w1124 w1135 w1146 w1164 w1170 w1264 _ w1276 w1314 _ w1384 w1389 w1393 w1404 w1409 w1433 _ w1441 _ _ _ _ _ w1577 _ w1594 w1609 w1635 w1638 w1661 w1721 _ w1738 w1741 _ _ _]
      tunnel: [w814 _ _ _ w842 _ _ w875 _ _ w918 _ w933 _ _ w996 w999 w1006 w1009 w1047 w1064 w1072 w1085 w1096 w1107 w1118 w1129 w1140 w1162 w1169 w1262 _ w1274 w1312 _ _ w1387 w1391 w1394 w1407 w1431 _ w1439 _ _ _ _ _ w1575 _ _ _ _ _ _ _ _ _ _ _ _ _] -> w773
      tunnel: w772 -> [w813 _ _ _ w851 _ _ w874 _ _ w918 _ w952 _ _ w995 w998 w1005 w1008 w1046 w1065 w1071 w1090 w1101 w1112 w1123 w1134 w1145 w1163 w1168 w1263 _ w1275 w1313 _ _ w1388 w1392 w1403 w1408 w1432 _ w1440 _ _ _ _ _ w1576 _ w1593 w1608 w1634 w1637 w1662 w1720 _ w1737 _ _ _ _]
      tunnel: [_ _ _ _ _ _ _ _ _ _ w917 _ _ _ _ _ _ _ _ _ _ _ _ _ _ _ _ _ _ _ _ _ _ _ _ _ _ _ _ _ _ _ _ _ _ _ _ _ _ _ _ _ _ _ _ _ _ _ _ _ _ _] -> w771
      tunnel: [_ _ _ _ _ _ _ _ "Round T1 X" _ _ _ _ _ _ _ _ _ _ _ _ _ _ _ _ _ _ _ _ _ _ _ _ _ _ _ _ _ _ _ _ _ _ _ _ _ _ _ _ _ _ _ _ _ _ _ _ _ _ _ _ _] -> _
      tunnel: [_ _ _ "Adjust Scale\nto Mean" _ _ _ _ _ _ _ _ _ _ _ _ _ _ _ _ _ _ _ _ _ _ _ _ _ _ _ _ _ _ _ _ _ _ _ _ _ _ _ _ _ _ _ _ _ _ _ _ _ _ _ "Set SP to Reading" _ _ _ _ _ _] -> _
      tunnel: [_ _ _ _ _ _ _ _ _ "Round T2 X" _ "Delayed Interlace Start" _ _ _ _ _ _ _ _ _ _ _ _ _ _ _ _ _ _ _ _ _ _ _ _ _ _ _ _ _ _ _ _ _ _ _ _ _ _ _ _ _ _ _ _ _ _ _ _ _ _] -> _
      event "AI Count (ticks)", "Sets to FIFO (Traps)", "Save ave N", "FPGA Ave.", "# Samples/channel", "N sets to save": Value Change {
        # "So that if 'Save ave N' is updated, the AOD scanning code updates too."
        n423 = event-data() -> ()  [unwired: 6 out]
        n424 = local read "AI Count (ticks)"() -> (w796:u32)
        n425 = Unbundle By Name("Sets to FIFO (Traps)") -> ("Set 1"=w779:bool, "Set 2"=w778:bool, "Set 3"=w777:bool)
        n426 = Boolean To (0,1)(Boolean="Sets to FIFO (Traps)") -> (0, 1=w805:cluster{"Set 1":i16, "Set 2":i16, "Set 3":i16})
        n427 = xnode "Read/Write Control"("FPGA VI Reference In"=w815, "error in"=w813, "ai count"=w796, "Set 1"=w779, "Set 2"=w778, "Set 3"=w777, "N of AI1 Int Acq Sets"="N Acq Sets (Traps + Fl.)") -> ("error out"=w814:errorcluster)  [unwired: 1 out]
        n428 = Cluster To Array(cluster=w805) -> (array=w804:i16[])
        n429 = To Unsigned Long Integer(number=w804) -> (unsigned 32bit integer=w785:u32[])
        n430 = local read "Scan steps (AOD)"() -> (w806:u64)
        n431 = Multiply(x=w796, y="N Acq Sets (Traps + Fl.)") -> (x*y=w794:u32)
        n432 = Divide(x=40000000.0, y=w796) -> (x/y=w788:dbl)
        "AI rate (Hz)" <- w788
        "Ave. Rate (Hz)" <- w788
        n433 = Add Array Elements(numeric array=w785) -> (sum=w797:u32)
        "Trap Sets" <- w797
        n434 = Reciprocal(x=w788) -> (1/x=→"Ave. Period (s)":dbl)
        n435 = property on="Scan steps (AOD)" class="DigNum (strict)"("Val(Sgnl)"=w806) -> ()  [unwired: 2 in, 2 out]
        n436 = Divide(x=w788, y="N Acq Sets (Traps + Fl.)") -> (x/y=w810:dbl)
        "Data Rate (Hz)" <- w810
        n437 = Reciprocal(x=w810) -> (1/x=→"Data Period (s)":dbl)
        n438 = local read "Save ave N"() -> (w809:dbl)
        n439 = Divide(x=w810, y=w809) -> (x/y=w808:dbl)
        "Save Data Rate (Hz)" <- w808
        n440 = Reciprocal(x=w808) -> (1/x=→"Save Data Period (s)":dbl)
        n441 = Multiply(x=w794, y="# Samples/trap") -> (x*y=w792:u32)
        "Counts/DMA" <- w792
        n442 = property on="Trap Disp. Downsample" class="DigNum (strict)"("Maximum"="# Samples/trap") -> ()  [unwired: 2 in, 2 out]
        n443 = Multiply(x=w797, y="# Samples/trap") -> (x*y=w786:u32)
        "# Samples/channel" <- w786
        n444 = Multiply(x=w786, y=u32 8) -> (x*y=→"Trap AI Elements/DMA read":u32)
        n445 = local read "APD Int. Count"() -> (w793:u32)
        n446 = Multiply(x=w786, y=u32 3) -> (x*y=→"Trap Pos Elements/DMA read":u32)
        n447 = Divide(x=w792, y=w793) -> (x/y=w783:dbl)
        "APD Samples/FIFO Acq." <- w783
        n448 = Divide(x=w792, y=40000000.0) -> (x/y=w790:dbl)
        "DMA Update Period (s)" <- w790
        n449 = Multiply(x=2.0, y=w783) -> (x*y=→"APD Elements/DMA read":dbl)
        n450 = property on="APD Disp. Downsample" class="DigNum (strict)"("Maximum"=w783) -> ()  [unwired: 2 in, 2 out]
        n451 = local read "N sets to save"() -> (w802:u32)
        n452 = Multiply(x=w790, y=w802) -> (x*y=→"Total Time (s)":dbl)
        "FPGA Averaging" <- FALSE ("FPGA Averaging")
      }
      event "Rescale on Mean": Value Change {
        n453 = event-data() -> ()  [unwired: 7 out]
        n454 = And(x=FALSE, y="Rescale on Mean") -> (x .and. y?=w817:bool)
        n455 = local write "Rescale on Mean"(w817) -> ()
        n456 = local read "Bead Mean (nm)"() -> (w822:dbl)
        n457 = Add(x="Amplitude (nm)", y=w822) -> (x+y=w820:dbl)
        n458 = Subtract(x=w822, y="Amplitude (nm)") -> (x-y=w819:dbl)
        n459 = property on="Bead Separation" class="WFChart (strict)"("YScale.Minimum"=w819) -> ()  [unwired: 2 in, 2 out]
        n460 = property on="Bead Separation" class="WFChart (strict)"("YScale.Maximum"=w820) -> ()  [unwired: 2 in, 2 out]
      }
      event "Detector Type": Value Change {
        n461 = event-data() -> ()  [unwired: 7 out]
        n462 = local read "AI labels"() -> (w823:string[])
        n463 = property on="High Res. Display" class="Ring (strict)"("Strings []"=w823) -> ()  [unwired: 2 in, 2 out]
        n464 = Build Array (concatenate)(w823, "none") -> (w824:string[])
        n465 = property on="FFT 1 Choice 1" class="Ring (strict)"("Strings []"=w824) -> ()  [unwired: 2 in, 2 out]
        n466 = property on="FFT 1 Choice 2" class="Ring (strict)"("Strings []"=w824) -> ()  [unwired: 2 in, 2 out]
        n467 = property on="FFT 2 Choice 1" class="Ring (strict)"("Strings []"=w824) -> ()  [unwired: 2 in, 2 out]
        n468 = property on="FFT 2 Choice 2" class="Ring (strict)"("Strings []"=w824) -> ()  [unwired: 2 in, 2 out]
        n469 = Bundle("APD 1", "APD 2") -> (w827:cluster{string, string})  [unwired: 1 out]
        n470 = Cluster To Array(cluster=w827) -> (array=w825:string[])
        n471 = Build Array (concatenate)(w825, w824) -> (w829:string[])
        n472 = Array Size(array=w829) -> (size(s)=w830:i32)
        n473 = property on="Signals to Plot" class="LstBox (strict)"("Item Names"=w829) -> ()  [unwired: 2 in, 2 out]
        n474 = property on="Signals to Plot" class="LstBox (strict)"("Number of Rows"=w830) -> ()  [unwired: 2 in, 2 out]
        n475 = property on="All Signals" class="WFChart (strict)"("LegNumRows"=w830) -> ()  [unwired: 2 in, 2 out]
      }
      event "Adjust Scale\nto Mean": Value Change {
        n476 = event-data() -> ()  [unwired: 7 out]
        n477 = local read "APD 1 Rate (Hz)"() -> (w839:dbl)
        n478 = Multiply(x=1000.0, y="Above (kHz)") -> (x*y=w837:dbl)
        n479 = Multiply(x=1000.0, y="Below (kHz)") -> (x*y=w835:dbl)
        n480 = Add(x=w837, y=w839) -> (x+y=w832:dbl)
        n481 = Subtract(x=w839, y=w835) -> (x-y=w833:dbl)
        n482 = property on="APD Chart" class="WFChart (strict)"("YScale.Minimum"=w833) -> ()  [unwired: 2 in, 2 out]
        n483 = property on="APD Chart" class="WFChart (strict)"("YScale.Maximum"=w832) -> ()  [unwired: 2 in, 2 out]
      }
      event "Phase adj. (AI1)", "+ phase (AI1)", "- phase (AI1)": Value Change {
        n484 = event-data() -> ()  [unwired: 7 out]
